vi "Set Message Class Icon.vi"(8 "error in (no error)":errorcluster, 10 "References":T1) -> (0 "error out":errorcluster)   [LabVIEW 2023, in "Message Maker.lvclass"]
doc: "Gets the icon from the Actor class, clears it's text layer, then adds a new layer that contains the send icon Glyph. Sets this new icon to the new message class, then applys this icon to all owned items\n\nAuthor: Derek Trepanier\nCopyright: MGI 2015"
uses:
  Message Maker.lvclass
  Message Maker.lvclass/Message Maker.ctl
  <vilib>/LabVIEW Icon API/LabVIEW Icon API.lvlib
  <vilib>/LabVIEW Icon API/API_Text.ctl
  <vilib>/LabVIEW Icon API/lv_icon/Controls/Layer.ctl
  <vilib>/LabVIEW Icon API/lv_icon/Classes/Layer/Layer.lvclass
  <vilib>/LabVIEW Icon API/lv_icon/Controls/LayerType.ctl
  <vilib>/LabVIEW Icon API/lv_icon/Classes/Icon/Icon.lvclass
  Scripting Refs.ctl
panel:
  out "new picture":picture
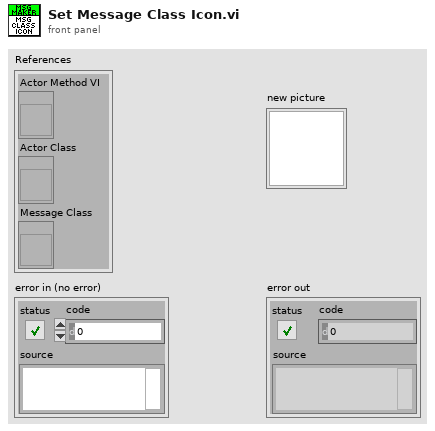
[diagram p1: front panel]
types:
  T1 = typedef "Message Maker.lvclass/Scripting Refs.ctl" = cluster{"Actor Method VI":refnum<vi>, "Actor Class":refnum<vi>, "Message Class":refnum<vi>}
  T2 = typedef "LayerType.ctl" = enum16{"Graphic", "Text", "Tool", "Graphic Drop"}
  T3 = typedef "Layer.ctl" = cluster{"LayerIcon":picture, "LayerName":string, "Opacity":u8, "Visibility?":bool}
  T4 = typedef "LabVIEW Icon API.lvlib/API_Text.ctl" = cluster{"Line 1 text":string, "Line 2 text":string, "Line 3 text":string, "Line 4 text":string}
  T5 = typedef "imagedata.ctl" = cluster{"image type":i32, "image depth":i32, "image":u8[], "mask":u8[], "colors":u32[], "Rectangle":cluster{"left":i16, "top":i16, "right":i16, "bottom":i16}}
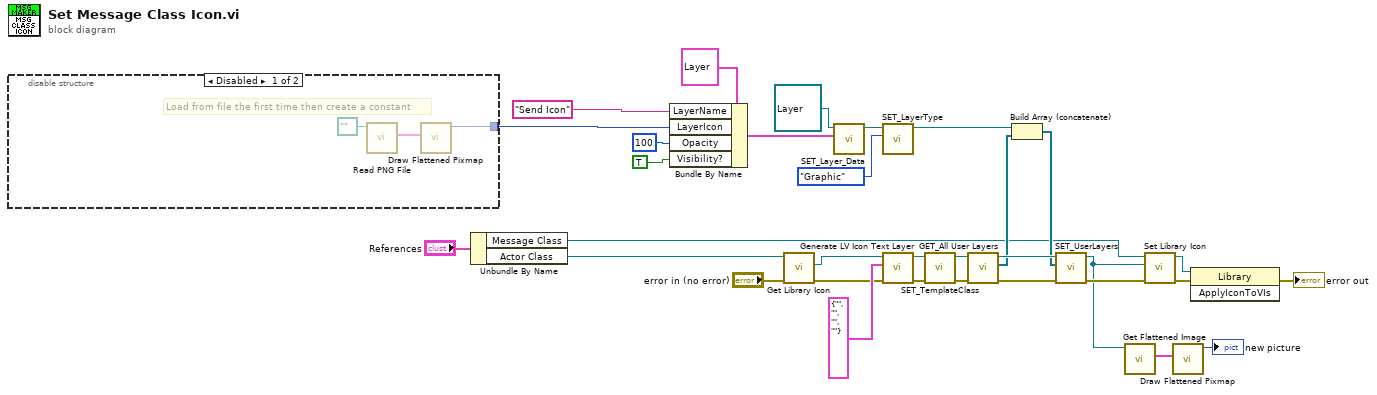
[diagram p0: block diagram]
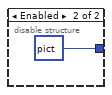
[diagram p2: hidden frame]
diagram:
  n1 = disable-structure shown="Disabled" {
    disable-tunnel: [w35 picture bytes[1182] ("new picture 2")] -> w7
    frame Disabled {
      # "Load from file the first time then create a constant"
      n2 = call <vilib>:"Read PNG File.vi"("path to PNG file"=path "") -> ("image data"=w34:T5)  [unwired: 8 in, 2 out]
      n3 = call <vilib>:"Draw Flattened Pixmap.vi"("image data"=w34) -> ("new picture"=w35:picture)  [unwired: 8 in]
    }
    frame Enabled {
    }
  }
  n4 = Unbundle By Name("References") -> ("Message Class"=w1:refnum<vi>, "Actor Class"=w2:refnum<vi>)
  n5 = Bundle By Name(cluster=T3 {"LayerIcon"=bytes[3102], "LayerName"="", "Opacity"=100, "Visibility?"=TRUE} ("Data"), "LayerName"="Send Icon", "LayerIcon"=w7, "Opacity"=u8 100, "Visibility?"=TRUE) -> (w13:T3)
  n6 = call <vilib>:"Get Library Icon.vi"("error in (no error)"="error in (no error)", "Library Refnum in"=w2) -> ("error out"=w19:errorcluster, "Icon"=w31:refnum<class "Icon.lvclass">)  [unwired: 7 in, 1 out]
  n7 = call-dynamic "SET_Layer_Data.vi"("Data"=w13, "Layer.lvclass in"=refnum<class "Layer.lvclass"> refnum) -> ("Layer.lvclass out"=w15:refnum<class "Layer.lvclass">)  [unwired: 2 in, 7 out]
  n8 = call-dynamic "SET_LayerType.vi"("Type"=LayerType."Graphic", "Layer.lvclass in"=w15) -> ("Layer.lvclass out"=w14:refnum<class "Layer.lvclass">)  [unwired: 1 in, 8 out]
  n9 = call <vilib>:"Generate LV Icon Text Layer.vi"("error in (no error)"=w19, "Text"=T4 {"Line 1 text"="", "Line 2 text"="", "Line 3 text"="", "Line 4 text"=""}, "Icon in"=w31) -> ("error out"=w20:errorcluster, "Icon out"=w28:refnum<class "Icon.lvclass">)  [unwired: 7 in]
  n10 = call-dynamic "SET_TemplateClass.vi"("error in (no error)"=w20, "Icon.lvclass in"=w28) -> ("error out"=w21:errorcluster, "Icon.lvclass out"=w27:refnum<class "Icon.lvclass">)  [unwired: 8 in]
  n11 = call-dynamic "GET_All User Layers.vi"("error in (no error)"=w21, "Icon.lvclass in"=w27) -> ("error out"=w22:errorcluster, "User Layer"=w29:refnum<class "Layer.lvclass">[], "Icon.lvclass out"=w30:refnum<class "Icon.lvclass">)  [unwired: 7 in]
  n12 = Build Array (concatenate)(w14, w29) -> (w23:refnum<class "Layer.lvclass">[])
  n13 = call-dynamic "SET_UserLayers.vi"("error in (no error)"=w22, "Layers"=w23, "Icon.lvclass in"=w30) -> ("error out"=w24:errorcluster, "Icon.lvclass out"=w6:refnum<class "Icon.lvclass">)  [unwired: 7 in]
  n14 = call <vilib>:"Get Flattened Image.vi"("lv_icon.lvlib:Icon.lvclass in"=w6) -> ("Color Image"=w5:T5)  [unwired: 7 in, 3 out]
  n15 = call <vilib>:"Set Library Icon.vi"("error in (no error)"=w24, "Icon"=w6, "Library Refnum in"=w1) -> ("error out"=w25:errorcluster, "Library Refnum out"=w26:refnum<vi>)  [unwired: 7 in]
  n16 = call <vilib>:"Draw Flattened Pixmap.vi"("image data"=w5) -> ("new picture"=→"new picture":picture)  [unwired: 8 in]
  n17 = invoke class="Library" method="ApplyIconToVIs"(reference=w26, error in=w25) -> (error out=→"error out":errorcluster)  [unwired: 1 in, 2 out]
